vi "myRIO_BRig_Host_TCP_parseCmd_trial__old.vi"(10 "input_countCmd":i32, 11 "input_strCmd":string) -> (1 "output_iState":i32, 2 "output_iTrial":i32, 3 "output_iBlock":i32, 4 "output_ai1":i32, 6 "output_ai0":i32)   [LabVIEW 2014]
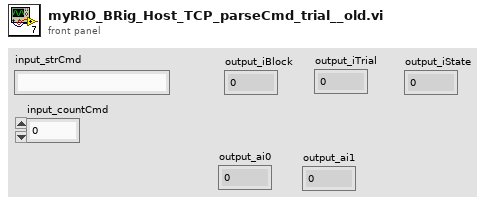
[diagram p1: front panel]
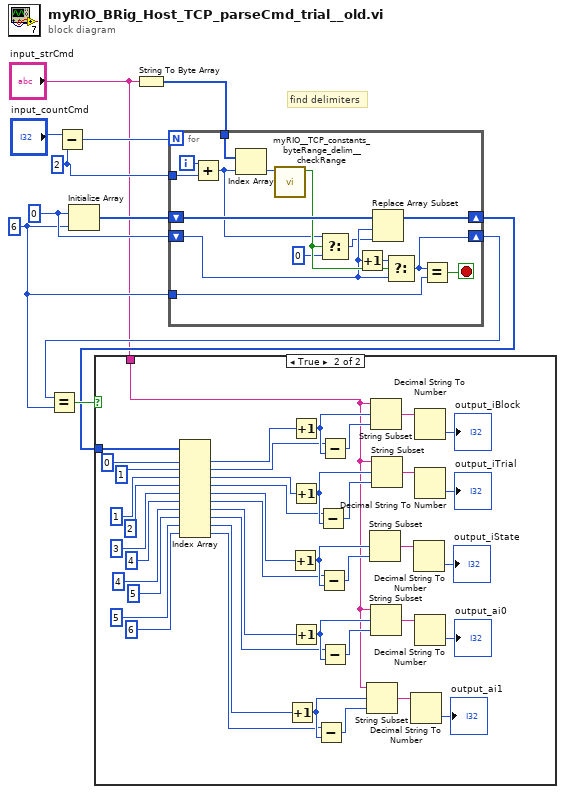
[diagram p0: block diagram]
diagram:
  w8 = 0 ("element")
  w2 = 6 ("dimension size")
  w9 = 2 ("y")
  # "find delimiters"
  n1 = Subtract(x="input_countCmd", y=w9) -> (x-y=w10:i32)
  n2 = Initialize Array(w8, w2) -> (w7:i32[])
  n3 = String To Byte Array(string="input_strCmd") -> (unsigned byte array=w6:u8[])
  n4 = for {
    N: w10 -> [_]
    tunnel: w9 -> [w25]
    shift-right: [w15] -> w5
    shift-left: w8 -> [w17]
    shift-right: [w12] -> w3
    shift-left: w7 -> [w24]
    tunnel: w6 -> [w23]
    tunnel: w2 -> [w14]
    i -> [w26]
    stop <- w13 stop-if-true
    n5 = Add(x=w26, y=w25) -> (x+y=w20:i32)
    n6 = Index Array(array=w23, index=w20) -> (element=w22:u8)
    n7 = call "myRIO__TCP_constants_byteRange_delim__checkRange.vi"("input_byte"=w22) -> ("output_delim"=w21:bool)  [unwired: 9 in, 1 out]
    n8 = Select(t=w20, s=w21, f=0) -> (s? t:f=w16:i32)
    n9 = Increment(x=w17) -> (x+1=w18:i32)
    n10 = Replace Array Subset(array=w24, new element=w16, index=w17) -> (w12:i32[])
    n11 = Select(t=w18, s=w21, f=w17) -> (s? t:f=w15:i32)
    n12 = Equal?(x=w15, y=w14) -> (x = y?=w13:bool)
  }
  n13 = Equal?(x=w5, y=w2) -> (x = y?=w4:bool)
  n14 = case shown="True" w4 {
    tunnel: w3 -> [_ w68]
    tunnel: "input_strCmd" -> [_ w29]
    frame False {
    }
    frame True {
      n15 = Index Array(array=w68, index #1=0 ("index"), index #2=1 ("index"), index #3=1 ("index"), index #4=2 ("index"), index #5=3 ("index"), index #6=4 ("index"), index #7=4 ("index"), index #8=5 ("index"), index #9=5 ("index"), index #10=6 ("index")) -> (element #1=w28:i32, element #2=w27:i32, element #3=w53:i32, element #4=w52:i32, element #5=w39:i32, element #6=w38:i32, element #7=w54:i32, element #8=w55:i32, element #9=w41:i32, element #10=w40:i32)
      n16 = Increment(x=w41) -> (x+1=w42:i32)
      n17 = Increment(x=w39) -> (x+1=w46:i32)
      n18 = Increment(x=w28) -> (x+1=w30:i32)
      n19 = Increment(x=w53) -> (x+1=w67:i32)
      n20 = Increment(x=w54) -> (x+1=w60:i32)
      n21 = Subtract(x=w40, y=w42) -> (x-y=w45:i32)
      n22 = Subtract(x=w52, y=w67) -> (x-y=w66:i32)
      n23 = Subtract(x=w38, y=w46) -> (x-y=w49:i32)
      n24 = Subtract(x=w27, y=w30) -> (x-y=w33:i32)
      n25 = Subtract(x=w55, y=w60) -> (x-y=w63:i32)
      n26 = String Subset(string=w29, offset (0)=w42, length (rest)=w45) -> (substring=w43:string)
      n27 = String Subset(offset (0)=w46, length (rest)=w49) -> (substring=w47:string)  [unwired: 1 in]
      n28 = String Subset(string=w29, offset (0)=w30, length (rest)=w33) -> (substring=w31:string)
      n29 = String Subset(string=w29, offset (0)=w60, length (rest)=w63) -> (substring=w61:string)
      n30 = String Subset(string=w29, offset (0)=w67, length (rest)=w66) -> (substring=w65:string)
      n31 = Decimal String To Number(string=w43) -> (number=→"output_ai1":i32)  [unwired: 2 in, 1 out]
      n32 = Decimal String To Number(string=w47) -> (number=→"output_iState":i32)  [unwired: 2 in, 1 out]
      n33 = Decimal String To Number(string=w31) -> (number=→"output_iBlock":i32)  [unwired: 2 in, 1 out]
      n34 = Decimal String To Number(string=w65) -> (number=→"output_iTrial":i32)  [unwired: 2 in, 1 out]
      n35 = Decimal String To Number(string=w61) -> (number=→"output_ai0":i32)  [unwired: 2 in, 1 out]
    }
  }
